vi "例8.7 连续输出(允许重生成)1.vi"() -> ()   [LabVIEW 2017]
uses:
  <vilib>/measure/NI_MABase.lvlib
panel:
  in  "sampling info":cluster{"Fs":dbl, "#s":dbl}={"Fs"=1000.0, "#s"=150.0} caption="采样信息" {"Fs" format="%.2p"}
  in  "amplitude":dbl=1.0 caption="幅值" format="%0.2p"
  in  "frequency":dbl=10.0 caption="频率" format="%0.2p"
  in  "停止":bool
  out "波形图":waveform(dbl)(graph)
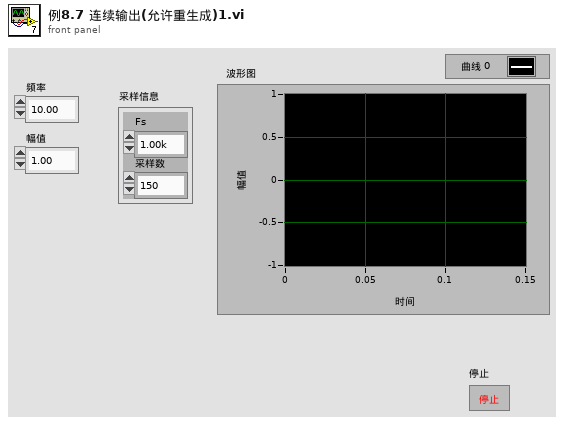
[diagram p1: front panel]
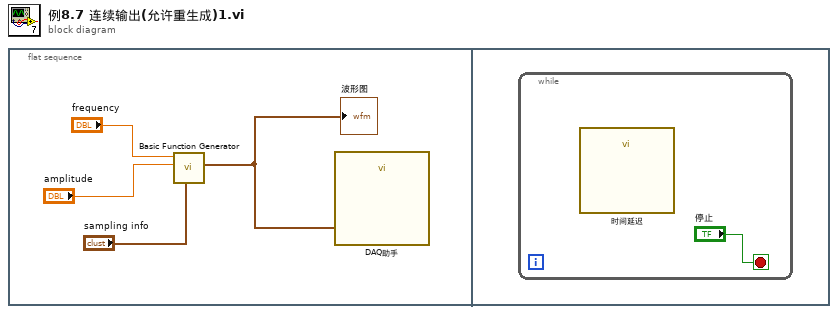
[diagram p0: block diagram]
diagram:
  n1 = flat-sequence {
    frame #0 {
      n2 = call <vilib>:"Basic Function Generator.vi"("sampling info"="sampling info", "amplitude"="amplitude", "frequency"="frequency") -> ("signal out"=w4:waveform(dbl))  [unwired: 6 in, 2 out]
      "波形图" <- w4
      n3 = call "DAQ助手"("data"=w4) -> ()  [unwired: 16 in, 3 out]
    }
    frame #1 {
      n4 = while {
        stop <- "停止" stop-if-true
        n5 = call "时间延迟"() -> ()  [unwired: 11 in, 1 out]
      }
    }
  }
